vi "Convert FLI Parameters v1 to v2.vi"(2 "FLI Parameters":T1) -> (7 "FLI Parameters v2":T2)   [LabVIEW 2021, in "Phasor.lvlib"]
uses:
  Phasor.lvlib
  Phasor Fluorescence Lifetime Parameters v2.ctl
  Fluorescence Lifetime Parameters.ctl
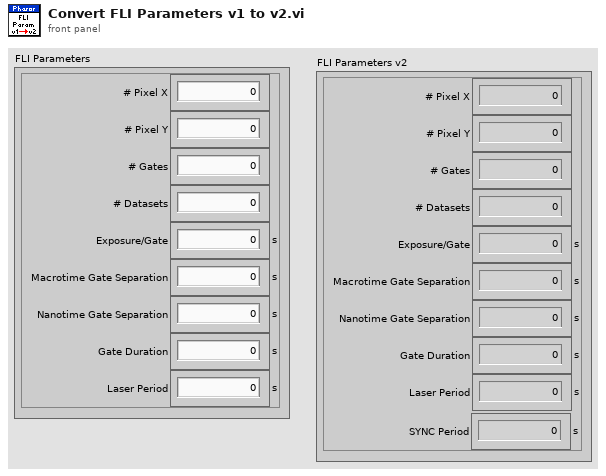
[diagram p1: front panel]
types:
  T1 = typedef "Phasor.lvlib/Fluorescence Lifetime Parameters.ctl" = cluster{"# Pixel X":i32, "# Pixel Y":i32, "# Gates":i32, "# Datasets":i32, "Exposure/Gate":dbl[unit], "Macrotime Gate Separation":dbl[unit], "Nanotime Gate Separation":dbl[unit], "Gate Duration":dbl[unit], "Laser Period":dbl[unit]}
  T2 = typedef "Phasor.lvlib/Phasor Fluorescence Lifetime Parameters v2.ctl" = cluster{"# Pixel X":i32, "# Pixel Y":i32, "# Gates":i32, "# Datasets":i32, "Exposure/Gate":dbl[unit], "Macrotime Gate Separation":dbl[unit], "Nanotime Gate Separation":dbl[unit], "Gate Duration":dbl[unit], "Laser Period":dbl[unit], "SYNC Period":dbl[unit]}
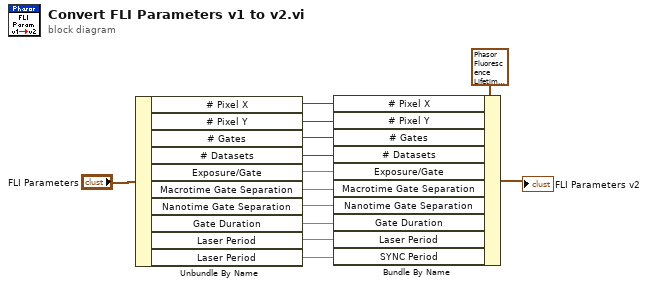
[diagram p0: block diagram]
diagram:
  n1 = Unbundle By Name("FLI Parameters") -> ("# Pixel X"=w12:i32, "# Pixel Y"=w10:i32, "# Gates"=w9:i32, "# Datasets"=w8:i32, "Exposure/Gate"=w7:dbl[unit], "Macrotime Gate Separation"=w6:dbl[unit], "Nanotime Gate Separation"=w5:dbl[unit], "Gate Duration"=w4:dbl[unit], "Laser Period"=w3:dbl[unit], "Laser Period"=w2:dbl[unit])
  n2 = Bundle By Name(cluster=T2 {"# Pixel X"=0, "# Pixel Y"=0, "# Gates"=0, "# Datasets"=0, "Exposure/Gate"=0.0, "Macrotime Gate Separation"=0.0, "Nanotime Gate Separation"=0.0, "Gate Duration"=0.0, "Laser Period"=0.0, "SYNC Period"=0.0} ("FLI Parameters v2"), "# Pixel X"=w12, "# Pixel Y"=w10, "# Gates"=w9, "# Datasets"=w8, "Exposure/Gate"=w7, "Macrotime Gate Separation"=w6, "Nanotime Gate Separation"=w5, "Gate Duration"=w4, "Laser Period"=w3, "SYNC Period"=w2) -> (→"FLI Parameters v2":T2)
